vi "failIfEqual.vi"(6 "delta (optional)":variant, 7 "custom report message (\"\")":string, 8 "error in (no error)":errorcluster, 9 "y":variant, 10 "x":variant, 11 "TestCase in":refnum<class "TestCase.lvclass">) -> (0 "error out":errorcluster, 3 "TestCase out":refnum<class "TestCase.lvclass">)   [LabVIEW 2013, in "TestCase.lvclass"]
doc: "Fail test if 'x' = 'y'. 'delta (optional)' if specified must be a numeric format and forces 'x', 'y' to be numeric. If 'delta' is not specified, x,y can be any variant data."
uses:
  TestCase.lvclass
  TestCase.lvclass/TestCase.ctl
  Libraries/VITesterUtilities.lvlib
panel:
  # "JKI VI Tester for LabVIEW\nhttp://jkisoft.com/vi-tester\nCopyright (C) 2007-2009, JKI <info@jkisoft.com>\nALL RIGHTS RESERVED"
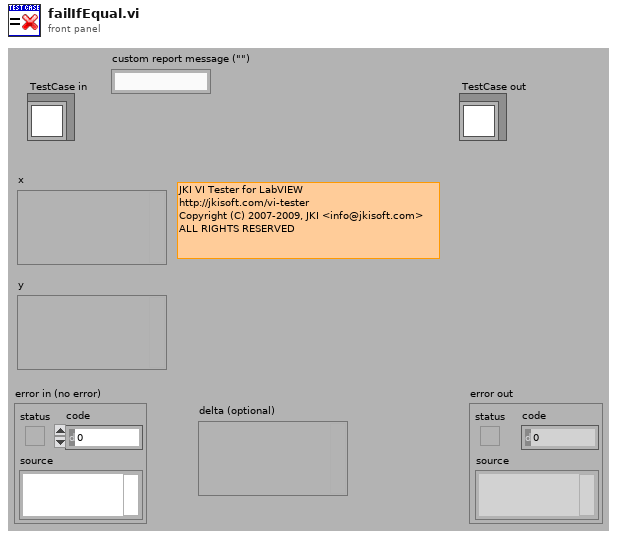
[diagram p1: front panel]
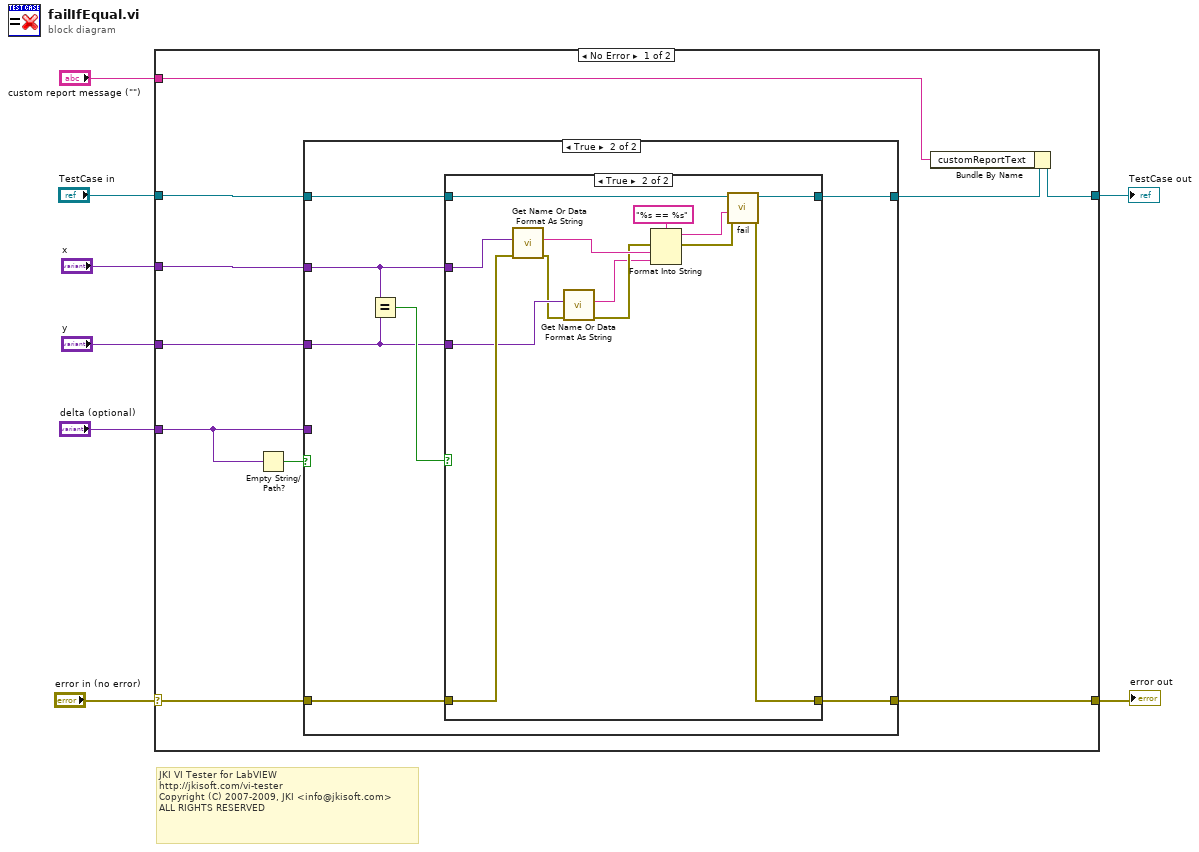
[diagram p0: block diagram]
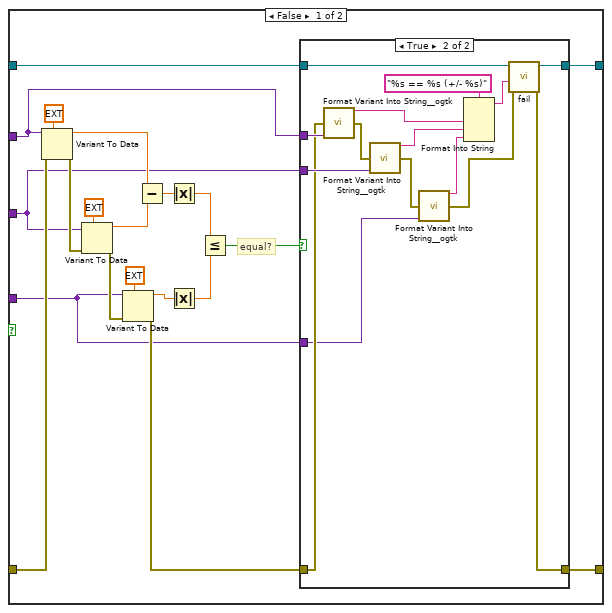
[diagram p2: hidden frame]
diagram:
  # "JKI VI Tester for LabVIEW\nhttp://jkisoft.com/vi-tester\nCopyright (C) 2007-2009, JKI <info@jkisoft.com>\nALL RIGHTS RESERVED"
  n1 = case shown="No Error" "error in (no error)" {
    selector: "error in (no error)" -> [w16 w79]
    tunnel: [w15 w79] -> w2
    tunnel: [w10 w78] -> w3
    tunnel: "TestCase in" -> [w13 w78]
    tunnel: "delta (optional)" -> [w14 _]
    tunnel: "x" -> [w18 _]
    tunnel: "y" -> [w12 _]
    tunnel: "custom report message (\"\")" -> [w9 _]
    frame No Error {
      n2 = Empty String/Path?(string/path=w14) -> (empty?=w17:bool)
      n3 = case shown="True" w17 {
        tunnel: w18 -> [w21 w57]
        tunnel: w12 -> [w20 w56]
        tunnel: w16 -> [w35 w61]
        tunnel: [w24 w60] -> w15
        tunnel: w14 -> [w19 _]
        tunnel: w13 -> [w23 w59]
        tunnel: [w22 w58] -> w11
        frame False {
          # "equal?"
          n4 = Variant To Data(error in=w35, type=ext 0.0, Variant=w21) -> (data=w32:ext, error out=w36:errorcluster)
          n5 = Variant To Data(error in=w36, type=ext 0.0, Variant=w20) -> (data=w31:ext, error out=w33:errorcluster)
          n6 = Variant To Data(error in=w33, type=ext 0.0, Variant=w19) -> (data=w29:ext, error out=w25:errorcluster)
          n7 = Subtract(x=w32, y=w31) -> (x-y=w30:ext)
          n8 = Absolute Value(x=w30) -> (abs(x)=w28:ext)
          n9 = Absolute Value(x=w29) -> (abs(x)=w27:ext)
          n10 = Less Or Equal?(x=w28, y=w27) -> (x <= y?=w26:bool)
          n11 = case shown="True" w26 {
            tunnel: [w40 w55] -> w24
            tunnel: w25 -> [w40 w49]
            tunnel: w23 -> [w39 w54]
            tunnel: [w39 w53] -> w22
            tunnel: w21 -> [_ w52]
            tunnel: w20 -> [_ w50]
            tunnel: w19 -> [_ w44]
            frame False {
            }
            frame True {
              n12 = call <userlib>:"Format Variant Into String__ogtk.vi"("error in (no error)"=w49, "Variant"=w52) -> ("Output String"=w47:string, "error out"=w51:errorcluster)  [unwired: 12 in]
              n13 = call <userlib>:"Format Variant Into String__ogtk.vi"("error in (no error)"=w51, "Variant"=w50) -> ("Output String"=w48:string, "error out"=w42:errorcluster)  [unwired: 12 in]
              n14 = call <userlib>:"Format Variant Into String__ogtk.vi"("error in (no error)"=w42, "Variant"=w44) -> ("Output String"=w43:string, "error out"=w41:errorcluster)  [unwired: 12 in]
              n15 = Format Into String(format string="%s == %s (+/- %s)", w47, w48, w43) -> (resulting string=w45:string)  [unwired: 2 in, 1 out]
              n16 = call-dynamic "fail.vi"("error in (no error)"=w41, "message (\"\")"=w45, "TestCase in"=w54) -> ("error out"=w55:errorcluster, "TestCase out"=w53:refnum<class "TestCase.lvclass">)  [unwired: 7 in]
            }
          }
        }
        frame True {
          n17 = Equal?(x=w57, y=w56) -> (x = y?=w62:bool)
          n18 = case shown="True" w62 {
            tunnel: w61 -> [w63 w71]
            tunnel: [w63 w75] -> w60
            tunnel: w59 -> [w64 w74]
            tunnel: [w64 w73] -> w58
            tunnel: w57 -> [_ w70]
            tunnel: w56 -> [_ w68]
            frame False {
            }
            frame True {
              n19 = call "Get Name Or Data Format As String.vi"("error in (no error)"=w71, "Data"=w70) -> ("error out"=w67:errorcluster, "Data Value OR Name"=w69:string)  [unwired: 8 in]
              n20 = call "Get Name Or Data Format As String.vi"("error in (no error)"=w67, "Data"=w68) -> ("error out"=w66:errorcluster, "Data Value OR Name"=w65:string)  [unwired: 8 in]
              n21 = Format Into String(format string="%s == %s", error in=w66, w69, w65) -> (resulting string=w76:string, error out=w72:errorcluster)  [unwired: 1 in]
              n22 = call-dynamic "fail.vi"("error in (no error)"=w72, "message (\"\")"=w76, "TestCase in"=w74) -> ("error out"=w75:errorcluster, "TestCase out"=w73:refnum<class "TestCase.lvclass">)  [unwired: 7 in]
            }
          }
        }
      }
      n23 = Bundle By Name(cluster=w11, "customReportText"=w9) -> (w10:refnum<class "TestCase.lvclass">)
    }
    frame Error {
    }
  }
  "error out" <- w2
  "TestCase out" <- w3
